vi "Datetime string to timestamp.vi"(3 "timestamp string":string) -> (0 "time stamp":timestamp, 1 "Time in sec":dbl, 2 "Offset":dbl)   [LabVIEW 2012]
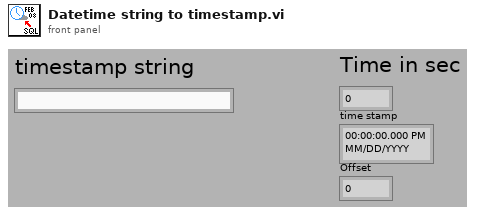
[diagram p1: front panel]
types:
  T1 = typedef "LVDateTimeRec.ctl" = cluster{"fractional second":dbl, "second":i32, "minute":i32, "hour":i32, "day of month":i32, "month":i32, "year":i32, "day of week":i32, "day of year":i32, "DST":i32}
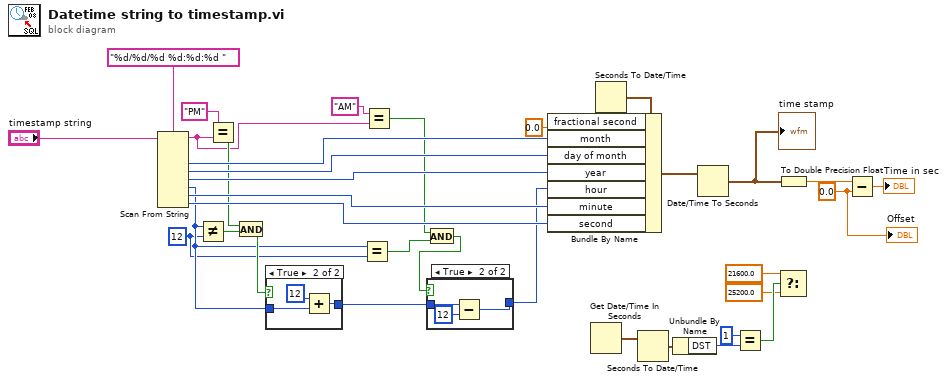
[diagram p0: block diagram]
diagram:
  w1 = 0.0 ("y")
  w11 = 12 ("y")
  n1 = Scan From String(format string="%d/%d/%d %d:%d:%d ", input string="timestamp string") -> (remaining string=w18:string, output 1=w28:i32, output 2=w27:i32, output 3=w26:i32, output 4=w12:i32, output 5=w30:i32, output 6=w29:i32)  [unwired: 2 in, 8 out]
  n2 = Not Equal?(x=w12, y=w11) -> (x != y?=w23:bool)
  n3 = Equal?(x="PM", y=w18) -> (x = y?=w24:bool)
  n4 = And(x=w24, y=w23) -> (x .and. y?=w22:bool)
  n5 = case shown="True" w22 {
    tunnel: w12 -> [w35 w37]
    tunnel: [w35 w38] -> w14
    frame False {
    }
    frame True {
      n6 = Add(x=12, y=w37) -> (x+y=w38:i32)
    }
  }
  n7 = Equal?(x=w12, y=w11) -> (x = y?=w16:bool)
  n8 = Equal?(x="AM", y=w18) -> (x = y?=w15:bool)
  n9 = And(x=w15, y=w16) -> (x .and. y?=w17:bool)
  n10 = case shown="True" w17 {
    tunnel: w14 -> [w39 w42]
    tunnel: [w39 w41] -> w13
    frame False {
    }
    frame True {
      n11 = Subtract(x=w42, y=12) -> (x-y=w41:i32)
    }
  }
  n12 = Get Date/Time In Seconds() -> (seconds since 1Jan1904=w10:timestamp)
  n13 = Seconds To Date/Time() -> (date time rec=w34:T1)  [unwired: 2 out]
  n14 = Bundle By Name(cluster=w34, "fractional second"=0.0, "month"=w28, "day of month"=w27, "year"=w26, "hour"=w13, "minute"=w30, "second"=w29) -> (w32:T1)
  n15 = Seconds To Date/Time(time stamp (now)=w10) -> (date time rec=w9:T1)  [unwired: 1 out]
  n16 = Unbundle By Name(w9) -> ("DST"=w6:i32)
  n17 = Date/Time To Seconds(2:w32) -> (0:w21:timestamp)  [unwired: 1 out]
  "time stamp" <- w21
  n18 = Equal?(x=1, y=w6) -> (x = y?=w4:bool)
  n19 = Select(t=21600.0, s=w4, f=25200.0) -> ()  [unwired: 1 out]
  n20 = To Double Precision Float(number=w21) -> (double precision float=w8:dbl)
  n21 = Subtract(x=w8, y=w1) -> (x-y=→"Time in sec":dbl)
  "Offset" <- w1
